vi "EXO3_2.vi"() -> ()   [LabVIEW 2019]
uses:
  <vilib>/myRIO/Instrument Drivers/Onboard Devices/Accelerometer/typedefs/Accelerometer Reference.ctl
  <vilib>/myRIO/Common/Instrument Driver Framework/Utilities/typedefs/myRIO Generic Hardware Reference.ctl
  <vilib>/myRIO/Common/Instrument Driver Framework/Utilities/typedefs/Hardware Version Enum.ctl
  <vilib>/myRIO/Common/Instrument Driver Framework/Utilities/typedefs/myRIO v1.0 Reference.ctl
  <vilib>/myRIO/Common/Instrument Driver Framework/Utilities/typedefs/Generic FPGA Reference.ctl
  <vilib>/myRIO/Common/Instrument Driver Framework/myRIO v1.0/Accelerometer/typedefs/Accelerometer Channels List.ctl
  <vilib>/myRIO/Common/Instrument Driver Framework/myRIO v1.0/Accelerometer/typedefs/Accelerometer Channels Enum.ctl
  <vilib>/userDefined/High Color/nirio_resource_hc.ctl
  <vilib>/myRIO/Instrument Drivers/Onboard IO/DIO/typedefs/DIO Reference.ctl
  <vilib>/myRIO/Common/Instrument Driver Framework/myRIO v1.0/DIO/typedefs/DIO Channels List.ctl
  <vilib>/myRIO/Common/Instrument Driver Framework/myRIO v1.0/DIO/typedefs/DIO Channels Enum.ctl
  <vilib>/myRIO/Common/Instrument Driver Framework/Utilities/vis/Is FPGA Ref Available.vi
  <vilib>/myRIO/Common/Instrument Driver Framework/myRIO v1.0/DIO/vis/myRIO v1.1 Open DIO.vi
  <vilib>/myRIO/Instrument Drivers/Onboard IO/DIO/vis/Read.vi
  <vilib>/myRIO/Common/Instrument Driver Framework/myRIO v1.0/Accelerometer/vis/myRIO v1.1 Open Accelerometer.vi
  <vilib>/myRIO/Instrument Drivers/Onboard Devices/Accelerometer/vis/Read.vi
  <vilib>/myRIO/Instrument Drivers/Onboard IO/DIO/vis/Write.vi
  <vilib>/myRIO/Common/Instrument Driver Framework/Utilities/vis/Validate Channels.vi
  <vilib>/myRIO/Common/Instrument Driver Framework/myRIO v1.0/DIO/vis/myRIO v1.0 Reserve DIO.vi
  <vilib>/myRIO/Common/Instrument Driver Framework/myRIO v1.0/Accelerometer/vis/myRIO v1.0 Reserve Accelerometer.vi
  <vilib>/myRIO/Common/Instrument Driver Framework/myRIO v1.0/Resource Manager/vis/myRIO v1.0 Reserve Channel List.vi
  <vilib>/myRIO/Common/Instrument Driver Framework/myRIO v1.0/DIO/vis/myRIO v1.0 Build MUX Configuration DIO.vi
  <vilib>/myRIO/Common/Instrument Driver Framework/myRIO v1.0/Accelerometer/vis/myRIO v1.0 Build MUX Configuration Accelerometer.vi
  <vilib>/myRIO/Common/Instrument Driver Framework/myRIO v1.0/Resource Manager/vis/myRIO v1.0 Reserve Channel.vi
  <vilib>/myRIO/Common/Instrument Driver Framework/myRIO v1.0/Resource Manager/vis/myRIO v1.0 Unreserve Channel.vi
  <vilib>/myRIO/Common/Instrument Driver Framework/myRIO v1.0/Resource Manager/vis/myRIO v1.0 Create Configuration List.vi
  <vilib>/myRIO/Common/Instrument Driver Framework/myRIO v1.0/Resource Manager/vis/myRIO v1.0 Build Mutex Name.vi
  <vilib>/Utility/VariantDataType/GetNumericInfo.vi
  <vilib>/Utility/error.llb/Error Cluster From Error Code.vi
  <vilib>/myRIO/Common/Instrument Driver Framework/myRIO v1.0/myRIO v1.1 Open.vi
  <vilib>/myRIO/Common/Instrument Driver Framework/myRIO v1.0/Accelerometer/vis/myRIO v1.0 Get Scaling Constant Accelerometer.vi
  <vilib>/myRIO/Common/Instrument Driver Framework/Utilities/vis/IO Manager.vi
  <vilib>/myRIO/Common/Instrument Driver Framework/Utilities/vis/Configuration Manager.vi
  <vilib>/myRIO/Common/Instrument Driver Framework/myRIO v1.0/myRIO v1.0 Close.vi
  <vilib>/myRIO/Common/Instrument Driver Framework/myRIO v1.0/Accelerometer/vis/myRIO v1.0 Read Accelerometer.vi
  <vilib>/myRIO/Common/Instrument Driver Framework/myRIO v1.0/Resource Manager/vis/myRIO v1.0 Configure IO.vi
  <vilib>/myRIO/Common/Instrument Driver Framework/myRIO v1.0/DIO/vis/myRIO v1.0 Write DIO.vi
  <vilib>/myRIO/Common/Instrument Driver Framework/myRIO v1.0/DIO/vis/myRIO v1.0 Read DIO.vi
  <vilib>/myRIO/Express VI/Onboard Devices/Accelerometer/Accelerometer Express VI.xnode
  <vilib>/myRIO/Instrument Drivers/Onboard Devices/Accelerometer/vis/myRIO Accelerometer Open.xnode
  <vilib>/myRIO/Express VI/Onboard Devices/LED/LED Express VI.xnode
  <vilib>/myRIO/Instrument Drivers/Onboard IO/DIO/vis/myRIO DIO Open.xnode
  <vilib>/myRIO/Express VI/Onboard Devices/Button/Button Express VI.xnode
  <vilib>/myRIO/Instrument Drivers/Onboard Devices/Accelerometer/Accelerometer.lvlib
  <vilib>/myRIO/Instrument Drivers/Onboard IO/DIO/DIO.lvlib
panel:
  out "Setpoint":string
  in  "?":bool
  out "Inclinaison en degré":dbl
  out "Z":dbl
  out "Y":dbl
  out "X":dbl
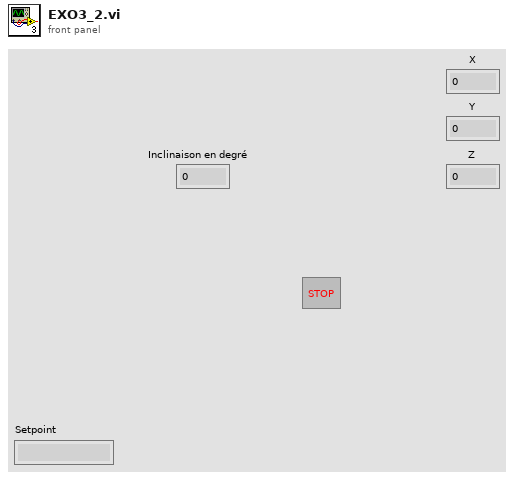
[diagram p1: front panel]
types:
  T1 = enum16{"open", "replace", "create", "open or create", "replace or create", "replace or create with confirmation"}
  T2 = typedef "DIO.lvlib/DIO Reference.ctl" = cluster{"myRIO Reference":T3, "DIO Channels List":T7}
  T3 = typedef "myRIO Generic Hardware Reference.ctl" = cluster{"myRIO Model":T4, "myRIO Hardware Reference":T5}
  T4 = typedef "Hardware Version Enum.ctl" = enum16{"Unknown", "myRIO-1900", "myRIO-1950", "roboRIO", "NI ELVIS RIO CM", "ELVIS III"}
  T5 = typedef "myRIO v1.0 Reference.ctl" = cluster{"Generic FPGA Reference":T6, "Allow multiple opens":bool}
  T6 = typedef "Generic FPGA Reference.ctl" = refnum<k20>
  T7 = typedef "DIO Channels List.ctl" = T8[]
  T8 = typedef "DIO Channels Enum.ctl" = enum16{"Not Connected", "C/DIO0", "C/DIO1", "C/DIO2", "C/DIO3", "C/DIO4", "C/DIO5", "C/DIO6", "C/DIO7", "A/DIO0", "A/DIO1", "A/DIO2", "A/DIO3", "A/DIO4", "A/DIO5", "A/DIO6", "A/DIO7", "A/DIO8", "A/DIO9", "A/DIO10", "A/DIO11", "A/DIO12", "A/DIO13", "A/DIO14", "A/DIO15", "A/DIO16", "A/DIO17", "A/DIO18", "A/DIO19", "B/DIO0", "B/DIO1", "B/DIO2", "B/DIO3", "B/DIO4", "B/DIO5", "B/DIO6", "B/DIO7", "B/DIO8", "B/DIO9", "B/DIO10", "B/DIO11", "B/DIO12", "B/DIO13", "B/DIO14", "B/DIO15", "B/DIO16", "B/DIO17", "B/DIO18", "B/DIO19", "LED0", "LED1", "LED2", "LED3", "Button0", "DIO/DIO0", "DIO/DIO1", "DIO/DIO2", "DIO/DIO3", "DIO/DIO4", "DIO/DIO5", "DIO/DIO6", "DIO/DIO7", "DIO/DIO8", "DIO/DIO9", "SPI/CS0", "SPI/CS1", "SPI/CS2", "SPI/CS3", "LED RADIO (Green)", "LED RADIO (Red)", "LED COMM (Green)", "LED COMM (Red)", "LED MODE (Green)", "LED MODE (Red)"}
  T9 = typedef "nirio_resource_hc.ctl" = tag
  T10 = typedef "Accelerometer.lvlib/Accelerometer Reference.ctl" = cluster{"myRIO Reference":T3, "Accelerometer Channels List":T11, "LSB Weight":dbl}
  T11 = typedef "Accelerometer Channels List.ctl" = T12[]
  T12 = typedef "Accelerometer Channels Enum.ctl" = enum16{"Not Connected", "X-Axis", "Y-Axis", "Z-Axis"}
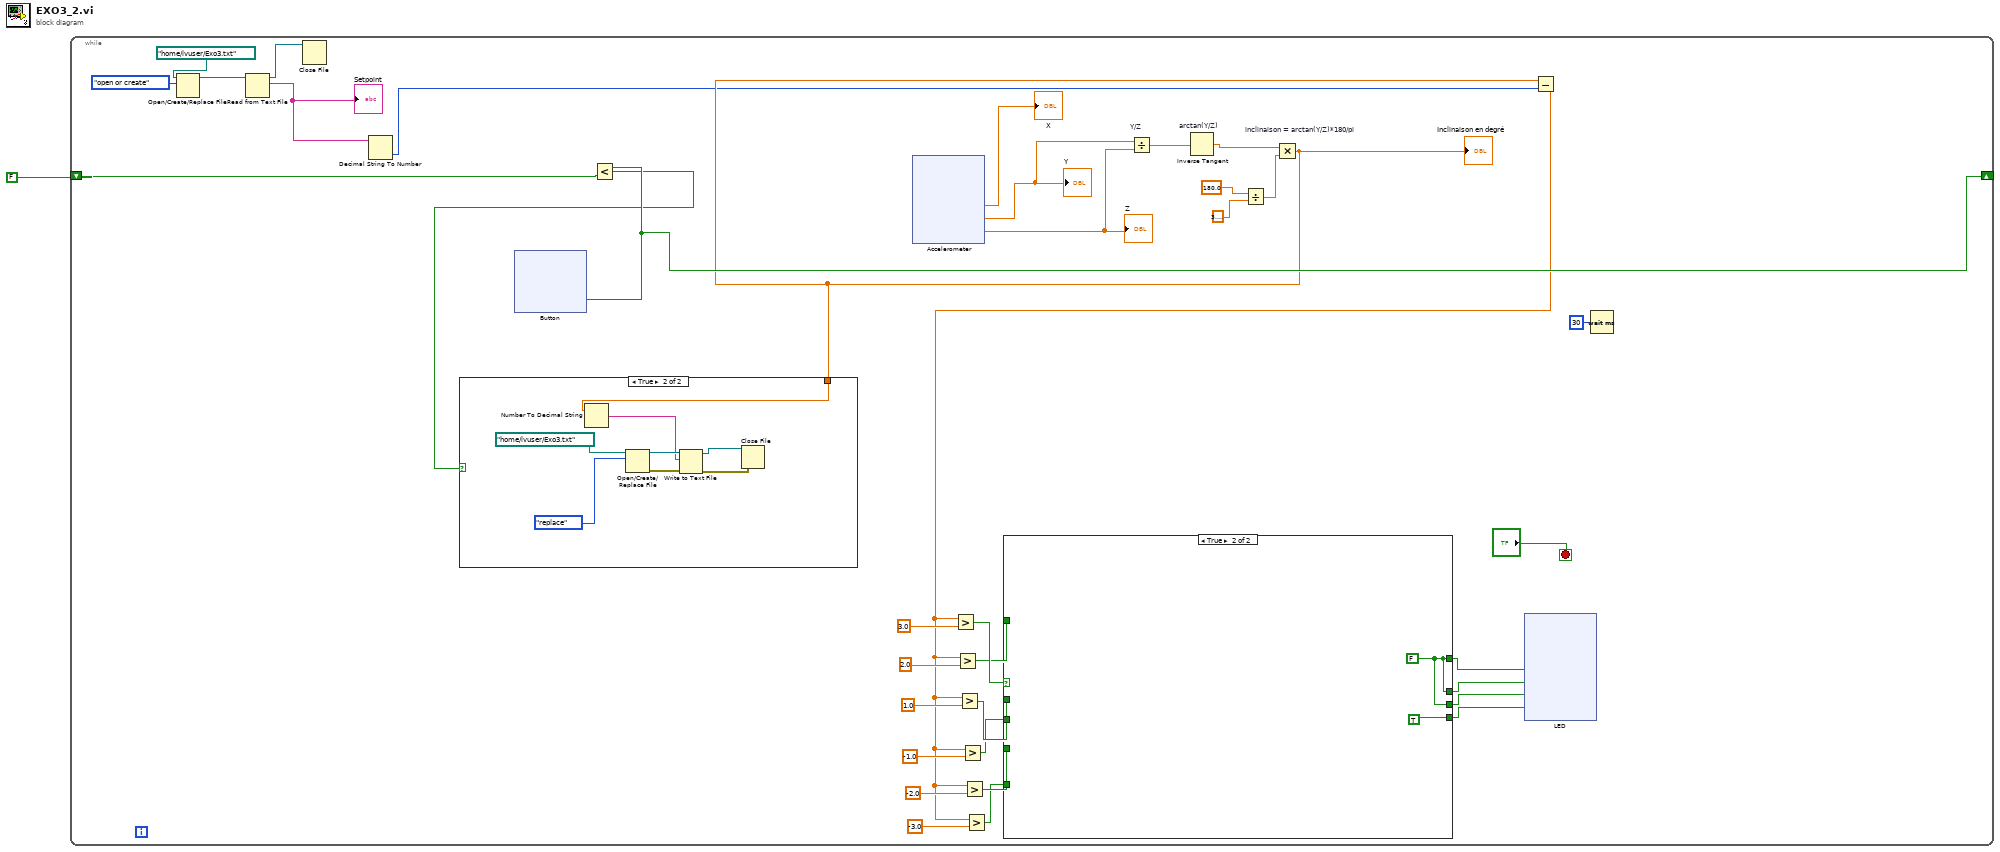
[diagram p0: block diagram]
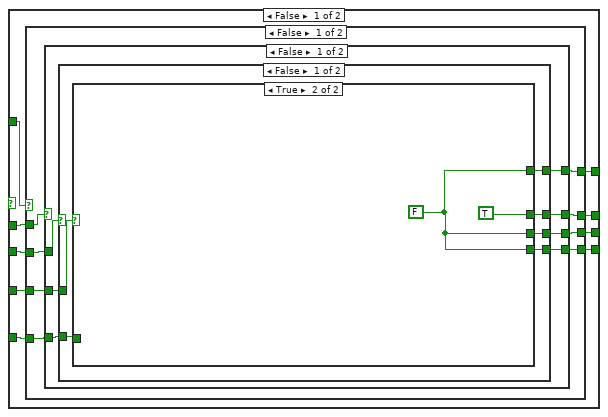
[diagram p3: hidden frame]
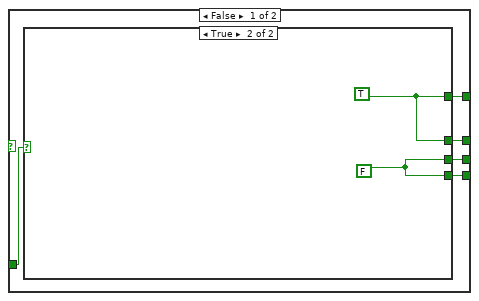
[diagram p4: hidden frame]
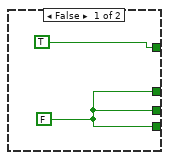
[diagram p5: hidden frame]
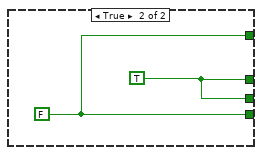
[diagram p6: hidden frame]
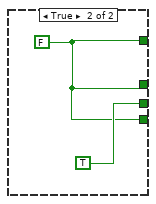
[diagram p7: hidden frame]
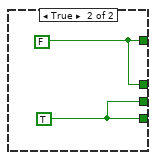
[diagram p8: hidden frame]
diagram:
  n1 = while {
    shift-right: [w12] -> _
    shift-left: FALSE -> [w14]
    stop <- "?" stop-if-true
    n2 = Open/Create/Replace File(file path (use dialog)=path "/home/lvuser/Exo3.txt", operation (0:open)=T1."open or create") -> (refnum out=w7:refnum<file>)  [unwired: 4 in, 2 out]
    n3 = Read from Text File(file (use dialog)=w7) -> (refnum out=w8:refnum<file>, text=w3:string)  [unwired: 3 in, 2 out]
    "Setpoint" <- w3
    n4 = Close File(refnum=w8) -> ()  [unwired: 1 in, 2 out]
    n5 = Decimal String To Number(string=w3) -> (number=w4:i32)  [unwired: 2 in, 1 out]
    n6 = xnode "Button"() -> ("Value"=w12:bool)  [unwired: 1 in, 1 out]
    n7 = Less?(x=w12, y=w14) -> (x < y?=w11:bool)
    n8 = xnode "Accelerometer"() -> ("X"=→"X":dbl, "Y"=w37:dbl, "Z"=w36:dbl)  [unwired: 1 in, 1 out]
    "Y" <- w37
    "Z" <- w36
    n9 = Divide "Y/Z"(x=w37, y=w36) -> (x/y=w35:dbl)
    n10 = Inverse Tangent "arctan(Y/Z)"(1:w35) -> (0:w32:dbl)
    n11 = Divide(x=180.0, y=3.141592653589793) -> (x/y=w31:dbl)
    n12 = Multiply "inclinaison = arctan(Y/Z)*180/pi"(x=w32, y=w31) -> (x*y=w10:dbl)
    "Inclinaison en degré" <- w10
    n13 = case shown="True" w11 {
      tunnel: w10 -> [_ w41]
      frame False {
      }
      frame True {
        n14 = Number To Decimal String(number=w41) -> (decimal integer string=w40:string)  [unwired: 1 in]
        n15 = Open/Create/Replace File(file path (use dialog)=path "/home/lvuser/Exo3.txt", operation (0:open)=T1."replace") -> (refnum out=w45:refnum<file>, error out=w43:errorcluster)  [unwired: 4 in, 1 out]
        n16 = Write to Text File(file (use dialog)=w45, text=w40, error in=w43) -> (refnum out=w44:refnum<file>, error out=w42:errorcluster)  [unwired: 1 in, 1 out]
        n17 = Close File(refnum=w44, error in=w42) -> ()  [unwired: 2 out]
      }
    }
    n18 = Subtract(x=w10, y=w4) -> (x-y=w9:dbl)
    n19 = Greater?(x=w9, y=3.0) -> (0:w24:bool)
    n20 = Greater?(x=w9, y=2.0) -> (0:w23:bool)
    n21 = Greater?(x=w9, y=1.0) -> (0:w22:bool)
    n22 = Greater?(x=w9, y=-1.0) -> (0:w20:bool)
    n23 = Greater?(x=w9, y=-2.0) -> (0:w18:bool)
    n24 = Greater?(x=w9, y=-3.0) -> (0:w16:bool)
    n25 = case shown="True" w24 {
      tunnel: [w88 w130] -> w2
      tunnel: [w87 w130] -> w30
      tunnel: [w89 w130] -> w29
      tunnel: [w90 TRUE] -> w28
      tunnel: w23 -> [w86 _]
      tunnel: w22 -> [w85 _]
      tunnel: w20 -> [w84 _]
      tunnel: w18 -> [w83 _]
      tunnel: w16 -> [w82 _]
      frame False {
        n26 = case shown="False" w86 {
          tunnel: [w95 w128] -> w90
          tunnel: [w98 w128] -> w89
          tunnel: [w97 w127] -> w88
          tunnel: [w96 w127] -> w87
          tunnel: w85 -> [w94 _]
          tunnel: w84 -> [w93 _]
          tunnel: w83 -> [w92 _]
          tunnel: w82 -> [w91 _]
          frame False {
            n27 = case shown="False" w94 {
              tunnel: [w103 TRUE] -> w98
              tunnel: [w102 w125] -> w97
              tunnel: [w104 w125] -> w96
              tunnel: [w101 w125] -> w95
              tunnel: w93 -> [w105 _]
              tunnel: w92 -> [w100 _]
              tunnel: w91 -> [w99 _]
              frame False {
                n28 = case shown="False" w105 {
                  tunnel: [w110 w124] -> w104
                  tunnel: [w107 w124] -> w103
                  tunnel: [w109 w123] -> w102
                  tunnel: [w108 w123] -> w101
                  tunnel: w100 -> [w111 _]
                  tunnel: w99 -> [w106 _]
                  frame False {
                    n29 = case shown="True" w111 {
                      tunnel: [w114 TRUE] -> w110
                      tunnel: [w115 w121] -> w109
                      tunnel: [w112 w121] -> w108
                      tunnel: [w113 w121] -> w107
                      tunnel: w106 -> [w116 _]
                      frame False {
                        n30 = case shown="True" w116 {
                          tunnel: [TRUE w120] -> w115
                          tunnel: [w117 w120] -> w114
                          tunnel: [w117 w119] -> w113
                          tunnel: [w117 w119] -> w112
                          frame False {
                            w117 = FALSE
                          }
                          frame True {
                            w120 = TRUE
                            w119 = FALSE
                          }
                        }
                      }
                      frame True {
                        w121 = FALSE
                      }
                    }
                  }
                  frame True {
                    w124 = TRUE
                    w123 = FALSE
                  }
                }
              }
              frame True {
                w125 = FALSE
              }
            }
          }
          frame True {
            w127 = FALSE
            w128 = TRUE
          }
        }
      }
      frame True {
        w130 = FALSE
      }
    }
    n31 = xnode "LED"("LED0"=w2, "LED1"=w30, "LED2"=w29, "LED3"=w28) -> ()  [unwired: 1 in, 1 out]
    n32 = Wait (ms)(milliseconds to wait=u32 30) -> ()  [unwired: 1 out]
  }
